vi "Find Level with Jokers.vi"(11 "Card":T2[](array[typedef])) -> (3 "Level":T1)   [LabVIEW 2023]
uses:
  ENUM_Joker Card.ctl
  ENUM_Level.ctl
  <vilib>/Utility/miscctls.llb/LVMapReplaceAction.ctl
panel:
  out "Joker count":i32
  out "sorted array":cluster{"Numeric":i32, "Card":T2}[](array[cluster])
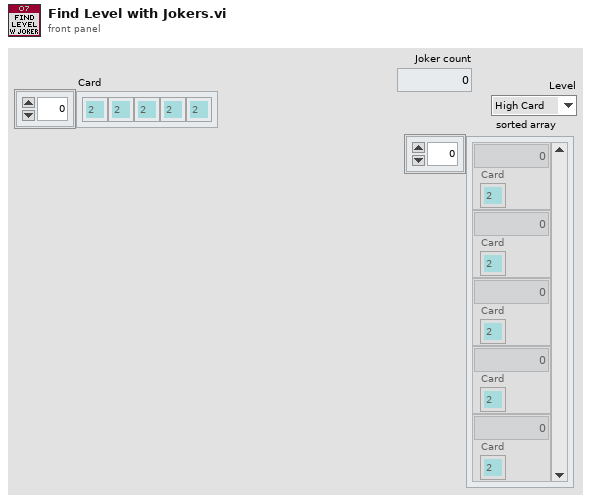
[diagram p1: front panel]
types:
  T1 = typedef "ENUM_Level.ctl" = enum16{"High Card", "One Pair", "Two Pair", "3 of a Kind", "Full House", "4 of a Kind", "5 of a Kind"}
  T2 = typedef "ENUM_Joker Card.ctl" = enum16{"J", "2", "3", "4", "5", "6", "7", "8", "9", "T", "Q", "K", "A"}
  T3 = typedef "LVMapReplaceAction.ctl" = enum32{"Modify Entry only if found", "Add or Modify Entry", "Delete Entry"}
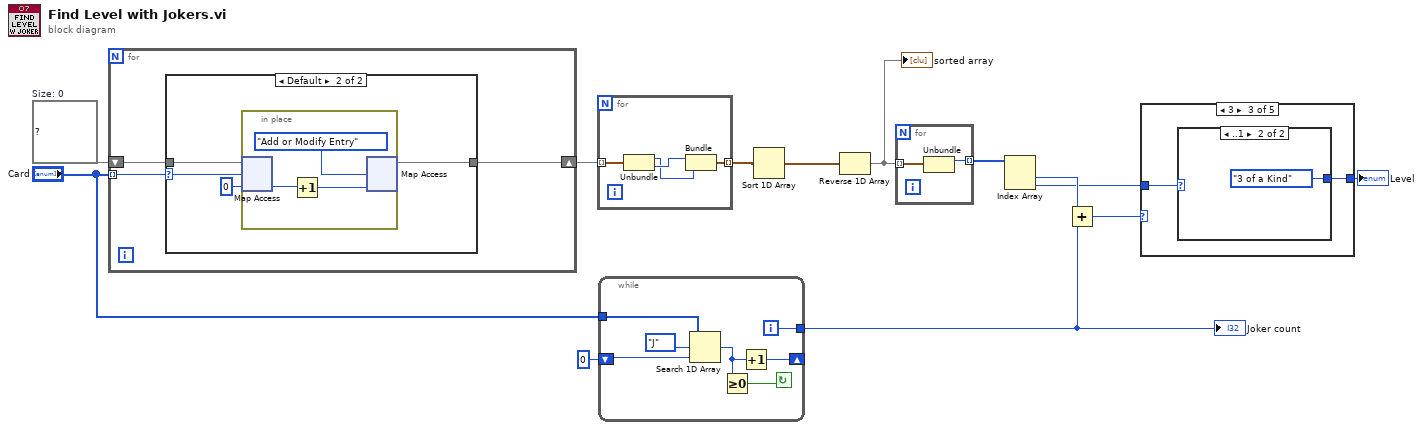
[diagram p0: block diagram]
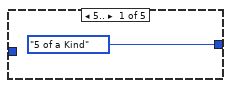
[diagram p2: hidden frame]
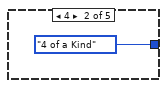
[diagram p3: hidden frame]
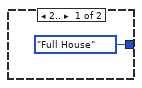
[diagram p4: hidden frame]
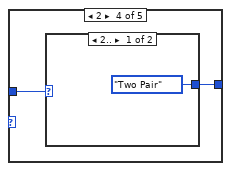
[diagram p5: hidden frame]
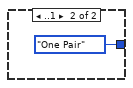
[diagram p6: hidden frame]
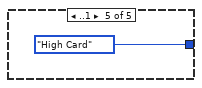
[diagram p7: hidden frame]
diagram:
  w13 = map{T2, i32} {}  # Size: 0
  n1 = for {
    tunnel: "Card" -> [w14] mode=indexing
    shift-right: [w15] -> w12
    shift-left: w13 -> [w16]
    n2 = case shown="Default" w14 {
      selector: w14 -> [_ w19]
      tunnel: w16 -> [w17 w21]
      tunnel: [w17 w20] -> w15
      frame "J" {
      }
      frame Default {
        n3 = in-place {
          n4 = in-place-map #1(w21, w19, 0) -> (w23:i32)  [unwired: 1 out]
          n5 = Increment(x=w23) -> (x+1=w22:i32)
          n6 = in-place-map #1(w22, LVMapReplaceAction."Add or Modify Entry" ("action")) -> (w20:map{T2, i32})  [unwired: 2 out]
        }
      }
    }
  }
  n7 = for {
    tunnel: w12 -> [w28] mode=indexing
    tunnel: [w25] -> w11 mode=indexing
    n8 = Unbundle(w28) -> ("Card"=w26:T2, w27:i32)
    n9 = Bundle(w27, "Card"=w26) -> (w25:cluster{i32, "Card":T2})  [unwired: 1 in]
  }
  n10 = while {
    tunnel: "Card" -> [w35]
    tunnel: [w32] -> w2
    shift-right: [w29] -> _
    shift-left: 0 ("index of element") -> [w30]
    i -> [w32]
    stop <- w33 continue-if-true
    n11 = Search 1D Array(1D array=w35, element=ENUM_Joker_Card."J" ("Card"), start index (0)=w30) -> (index of element=w31:i32)
    n12 = Greater Or Equal To 0?(x=w31) -> (x >= 0?=w33:bool)
    n13 = Increment(x=w31) -> (x+1=w29:i32)
  }
  "Joker count" <- w2
  n14 = Sort 1D Array(array=w11) -> (sorted array=w10:cluster{i32, "Card":T2}[])
  n15 = Reverse 1D Array(array=w10) -> (reversed array=w8:cluster{i32, "Card":T2}[])
  "sorted array" <- w8
  n16 = for {
    tunnel: w8 -> [w37] mode=indexing
    tunnel: [w36] -> w9 mode=indexing
    n17 = Unbundle(w37) -> (w36:i32)  [unwired: 1 out]
  }
  n18 = Index Array(array=w9) -> (element #1=w7:i32, element #2=w5:i32)  [unwired: 2 in]
  n19 = Add(x=w7, y=w2) -> (x+y=w3:i32)
  n20 = case shown="3" w3 {
    tunnel: [ENUM_Level."5 of a Kind" ("rank") ENUM_Level."4 of a Kind" ("rank") w41 w45 ENUM_Level."High Card" ("rank")] -> w6
    tunnel: w5 -> [_ _ w40 w44 _]
    frame 5.. {
    }
    frame 4 {
    }
    frame 3 {
      n21 = case shown="..1" w40 {
        tunnel: [ENUM_Level."Full House" ("rank") ENUM_Level."3 of a Kind" ("rank")] -> w41
        frame 2.. {
        }
        frame ..1 {
        }
      }
    }
    frame 2 {
      n22 = case shown="2.." w44 {
        tunnel: [ENUM_Level."Two Pair" ("rank") ENUM_Level."One Pair" ("rank")] -> w45
        frame 2.. {
        }
        frame ..1 {
        }
      }
    }
    frame ..1 {
    }
  }
  "Level" <- w6
